vi "calculations.vi"(8 "Jump":dbl format="%#_13g", 10 "Sampling rate":dbl format="%#_13g", 11 "Force data":dbl[](array[numeric])=[2085.326104471059, 2046.9367015003631, 2066.134196083894, 2065.551002863692, 2042.2839241875834, 2031.815973261881, 2023.6720169084117, 2006.8033050654276, 2002.7369130850595, 1985.280219853559, 1978.8890352729054, 1960.2683496851575, 1959.6835604088506, 1957.3819106220842, 1923.0349587901856, 1913.1462109444237, 1900.9278823300624, 1886.9671563075658, 1876.4944172135492, 1866.6040733116827, 1852.0585580128793, 1840.4178364223535, 1822.9627392469579, 1821.2211398668746, 1802.019655143082, 1783.9829608035889, 1772.3446332972203, 1750.2319706407304, 1742.0872162592084, 1722.301740287161, 1696.1178974819888, 1697.8730633389619, 1655.9645503457439, 1664.1364376810463, 1625.7135175321514, 1601.2752642473242, 1582.656174715681, 1558.7971245107942, 1536.692442134828, 1525.0429422357263, 1494.2127063421933, 1479.661604847023, 1444.1642271357675, 1420.8939563474496, 1394.129314406232, 1368.5246746810008, 1342.9248231240833, 1315.573795850454, 1288.8075578531323, 1261.4613187478171, 1230.0375152694012, 1194.5457237545127, 1177.0866364388546, 1145.667621128753, 1111.9166309658945, 1088.6391779251053, 1054.3089846823063, 1023.4715665363022, 992.0461670017816, 964.7015239525717, 942.5976396046577, 910.5874507938302, 876.8284803504483, 851.81421609789, 817.483224827039, 790.1377837497765, 759.297971519615, 735.4413153988853, 706.9223056287473, 681.329636324301, 655.1433994349719, 626.0491767251549, 596.9581461275479, 581.2422542480781, 546.332857925339, 520.7346024245261, 500.3667312603289, 472.4357028787071, 440.43588843256015, 431.1239495825817, 406.10330110560443, 391.5601798909579, 364.20276839291023, 345.0076678935362, 329.87975740258264, 313.003065279075, 292.05838511909434, 278.0928709282835, 259.4673971722215, 243.7586875452231, 229.21077816226247, 213.49648233889715, 203.01895507656647, 178.00309476790346, 165.20396701749735, 156.47681744382552, 144.838489937457, 131.4505827704818, 110.50749866660588, 104.10194958101008, 121.00018846193156, 96.54437855995202, 86.06844735372628, 79.65731207176384, 64.53339172107218, 55.803050035191035, 47.657497625616884, 45.32951291312223, 39.511147187990154, 44.75669405760071, 32.52320291024451, 24.383236697036796, 27.296808713890815, 35.442361123464764, 17.400878615657593, 22.638445204744375, 14.490498711013087, 12.165706110727744, 7.510534713791018, 8.672931013933386, 12.170494279042012, 14.500075047641422, 2.2689779844423468, 12.75049538703473, 6.929735577745719, 4.60095283719889, 6.348138413648245, 5.182550001296365, 8.09612201815018, 11.004905866690132, 1.1041876001426418, 3.4393545651084954, 8.673729041985967, 10.995329530061595, 1.109773796509086, 6.928139521640963, 4.598558753041756, 1.110571824561464, -9.934188096924103, -2.9606083241208556, 2.853767260749333, 7.508140629633681, 12.753687499244243, 1.1113698526138422, 2.855363316853887, -1.2222010562472552, 2.857757401011021, 6.344946301438733, 2.8545652888017115, 5.765743221498595, 7.51292879794795, 3.4377585090039418, 9.843307594599738, -1.2206050001424988, 2.853767260749333, 2.8529692326969553, -1.2190089440379455, 1.1089757684569106, 8.097718074254937, -1.2094326074094082, 1.1089757684569106, 4.021749757258347, 1.6929670167113164, 9.841711538495185, 4.019355673101416, 3.4385565370561175, 4.020153701153592, 4.019355673101416, 3.4385565370561175, 6.344946301438733, 5.759358997079571, 1.6929670167113164, 26.15196903090016, -2.382203272232894, 2.8561613449064676, 4.596962696937, 1.6913709606067628, 4.603346921355822, -0.05421855973824068, 3.4409506212132515, 15.66406740388875, 2.270574040547103, 5.1897322537675645, 1.1025915440378857, 3.436960480951361, 2.855363316853887, 2.852171204644577, -0.05581461584279419, 6.348138413648245, -1.2214030281948771, 5.76654124955077, 2.855363316853887, 1.1081777404045325, 15.669653600255192, 4.603346921355822, 1.1081777404045325, 2.8561613449064676, 1.6905729325543848, 2.8529692326969553, 5.186540141558052, 1.1089757684569106, 5.191328309872321, 20.90562413323742, 1.6905729325543848, 3.4385565370561175, 3.435364424846808, 1.6913709606067628, 2.8561613449064676, 2.271372068599481, 3.4377585090039418, 0.524984520202302, -0.6350176957833369, -0.062198840261819, 1.1065816842997762, -1.2182109159855674, -0.05581461584279419, -0.6374117799404712, -1.2174128879331891, -0.05342053168586258, -34.9971320606764, -0.6374117799404712, 26.148776918690643, -3.5422054882183303, 2.2737661527564126, 4.60015480914631, -0.05421855973824068, 2.276160236913547, 2.8529692326969553, 2.855363316853887, 8.67213298588121, 7.505746545476749, -3.5469936565325986, 15.06890376290105, -4.131782932839585, -1.2174128879331891, 5.181751973243784, -0.05581461584279419, -1.2190089440379455, 2.271372068599481, -1.7998080800830416, 17.994446200540537, 15.654491067260414, 4.020951729206172, 4.020951729206172, 2.272170096651859, 2.8561613449064676, 2.2737661527564126, -0.055016587790618784, 5.767339277603352, 8.676123126142897, -3.544599572375464, 4.014567504787148, -1.802202164240176, -1.2190089440379455, -2.382203272232894, 4.020153701153592, 1.1089757684569106, 1.1113698526138422, -6.451787364810458, -3.5438015443230864, -5.289391064667887, 9.256124234135616, -2.96300240827799, 6.934523746059988, 4.019355673101416, 0.5265805763070582, 5.18334802934854, 3.4377585090039418, 1.6921689886589384, 1.6905729325543848, 7.506544573529127, 2.8561613449064676, 8.678517210300235, -1.8053942764494857, -2.380607216128138, 2.2737661527564126, 3.436960480951361, -0.6358157238357149, -1.7990100520306636, -0.6374117799404712, 0.5257825482546801, 6.926543465536207, -2.3790111600233814, 13.908901546915613, 6.348138413648245, 0.5265805763070582, 4.016961588944282, 2.8545652888017115, 3.436960480951361, 10.416924478173634, -1.2182109159855674, -1.2182109159855674, 6.925745437484031, -16.943679132083755, 0.5289746604639898, -0.05741067194755039, -1.2182109159855674, 5.764945193446015, -11.694142122211304, -2.968588604644434, -0.6334216396785807, 1.6953611008684508, 9.260114374397709, -0.6350176957833369, 4.021749757258347, 8.09133384983591, 1.6921689886589384, 4.019355673101416, 9.837721398233091, 0.5273786043592336, 9.261710430502262, -0.6374117799404712, -5.292583176877197, -5.287795008563131, 1.1089757684569106, 4.019355673101416, -1.8006061081354197, 1.109773796509086, -2.38379932833765, -7.621365917424431, 2.276958264965925, -1.7998080800830416, 4.020153701153592, 4.590578472518178, 0.5265805763070582, 2.8561613449064676, 2.270574040547103, -0.05421855973824068, 5.760955053184326, 0.524984520202302, -1.2182109159855674, 3.4377585090039418, -12.857336450406455, -2.9661945204872997, 1.1089757684569106, -1.2182109159855674, 1.6913709606067628, 0.5289746604639898, -7.618173805214918, 8.680911294457166, -7.6077994405342055, -9.956532882390285, 5.179357889086853, 4.022547785310726, 2.272170096651859, -0.05342053168586258, 4.020951729206172, 2.2737661527564126, 2.8561613449064676, 9.25452817803086, 1.6881788483972504, -0.6350176957833369, -1.215816831828433, -2.380607216128138, -1.2182109159855674, 0.5265805763070582, 0.5289746604639898, 1.6913709606067628, -4.127792792577492, -1.7998080800830416, 9.843307594599738, -0.05581461584279419, 4.603346921355822, -1.2190089440379455, 2.271372068599481, 2.270574040547103, -1.8006061081354197, 1.6937650447636945, 3.4393545651084954, 7.514524854052706, 6.927341493588788, 0.5281766324116117, -6.444605112339257, 0.5257825482546801, 0.5297726885163679, 0.5297726885163679, 1.6921689886589384, 0.5289746604639898, 1.6929670167113164, 5.769733361760283, -3.5438015443230864, -0.055016587790618784, 11.00889600695182, 8.677719182247655, 2.853767260749333, -1.2182109159855674, 1.6929670167113164, 5.761753081236705, -0.05342053168586258, 1.68418870813536, 1.6929670167113164, -2.382203272232894, 9.251336065821754, -6.459767645334036, 5.184146057401121, 2.2753622088611687, 3.4409506212132515, 1.1081777404045325, -7.03737466916962, -2.962204380225612, 22.076798741955745, -2.949435931387765, 15.084864323948409, 2.272170096651859, 2.2737661527564126, 4.60015480914631, -1.2182109159855674, 2.856959372958643, 0.5297726885163679, 10.428096870906522, 2.8545652888017115, -2.3830013002850694, -4.12539870842056, 19.16322672510193, 0.5257825482546801, 1.109773796509086, 1.110571824561464, 3.4377585090039418, 4.021749757258347, -2.382203272232894, 5.184944085453297, 2.853767260749333, 1.1025915440378857, 11.57692669415907, 2.853767260749333, 1.110571824561464, 2.8561613449064676, 4.018557645048835, 2.8585554290633994, 3.436960480951361, -0.6374117799404712, -0.05262250363348448, 5.763349137341258, -4.130186876734829, 3.4385565370561175, 2.270574040547103, 1.6913709606067628, 1.6913709606067628, -3.5469936565325986, -0.6342196677309587, 3.432172312637295, -0.05262250363348448, 14.5008730756938, 15.080874183686518, 15.66406740388875, 22.646425485268153, 32.53916347129166, 43.59908592577221, 52.32862958360097, 56.40699198475469, 72.70767314053133, 86.09238819529702, 131.51043487440893, 153.04150036680116, 150.70074720546867, 183.29732134870807, 218.8034773685396, 260.12720108545045, 306.114076479822, 393.4071189739525, 503.9752204247154, 660.5142367088027, 818.794852372973, 968.9394919641973, 1064.9748465649946, 1098.749777569424, 1076.653075473981, 1010.3174815886691, 913.1205287157817, 826.9771140729557, 746.6568533235761, 658.1806657999416, 612.7785796818771, 597.6498711628711, 602.8850436678008, 637.2056605739712, 671.5214893118275, 709.3308911745303, 723.8700222489149, 708.727747253019, 705.8173673483744, 671.4775977689474, 642.953001802443, 628.3835456620686, 627.7899780771857, 650.4786517014064, 688.8776310087303, 730.191778389013, 778.4978601873033, 840.2022235172494, 859.4172747179323, 901.9177592399285, 936.850298376186, 996.8162544382583, 1003.7842480146951, 1027.053720774961, 1039.2672612210083, 1049.7415963711292, 1062.538330037379, 1049.7296259503441, 1043.895299664165, 1112.5900013560138, 1148.6681782033143, 1185.9135395190717, 1219.6629336258254, 1244.6875722430643, 1265.056241435314, 1275.5329706695923, 1281.357720619143, 1295.9024378898941, 1304.0503843836257, 1320.930268619343, 1333.153385402018, 1370.9699695171923, 1402.3913789114513, 1425.0864367600905, 1447.7814946087303, 1468.7269727967632, 1476.8773133746517, 1503.0619542078764, 1522.2594487914075, 1536.2265590383226, 1550.1936692852385, 1576.9607053106129, 1604.3093385000846, 1647.945086368443, 1693.9072228931914, 1740.457340806456, 1786.4218714153612, 1805.6273462794165, 1825.4104281673065, 1827.73123062733, 1818.9793421840347, 1851.5735222431174, 1856.7791677101093, 1887.6062114914332, 1934.1491471522265, 1987.6760369505043, 2032.4725850629004, 2082.5226603254305, 2109.283312126386, 2124.984041472861, 2135.448002258302, 2128.4480875597706, 2123.201742662108, 2119.120986176797, 2113.8794294474487, 2124.9385538738766, 2130.7569195990086, 2124.358552765884, 2117.379386796714, 2113.324167209079, 2076.0851901177402, 2046.4117643279835, 2016.1679137668618, 1985.918477009374, 1963.2369856376245, 1942.8810848942126, 1939.987463578668, 1917.3067702349704, 1908.5891969979273, 1907.4483474551985, 1857.3847057157782, 1831.7968245796458, 1808.5281498474321, 1788.1674609357062, 1766.058788419478, 1749.1908746045467, 1741.6348996395936, 1734.0781266465879, 1727.683749953725, 1720.1261789326675, 1716.0581908961942, 1706.747050074268, 1693.9479223238618, 1676.4920271204137, 1670.0920642311842, 1663.1097061498049, 1653.220160275991, 1652.6377650838408, 1655.5505390726426, 1656.7209156533086, 1654.9809123293305, 1664.8728522873018, 1656.1401165172638, 1652.068936368581, 1645.0849822310975, 1639.8474156420102, 1647.414562999697, 1639.8410314175912, 1640.426618721951, 1647.9865838271655, 1652.650533532679, 1656.1425106014208, 1648.5673829632108, 1639.2554441132324, 1641.5834288257267, 1641.58103474157, 1635.7642650725425, 1641.0002356055245, 1610.7172816698373]) -> (0 "Peak landing force":dbl, 1 "Peak force":dbl, 2 "flight time":dbl, 3 "Jump height":dbl)   [LabVIEW 2014]
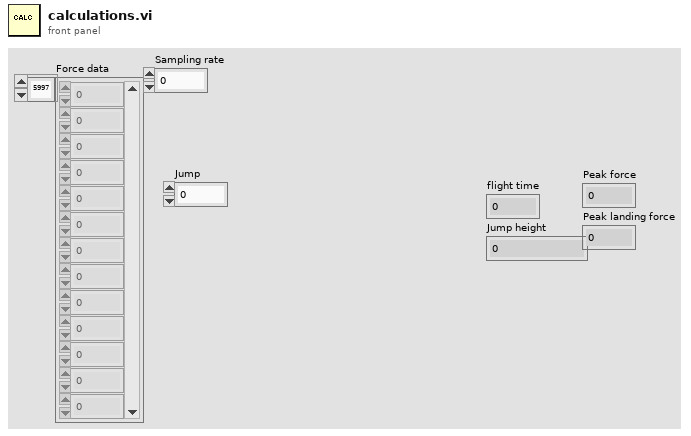
[diagram p1: front panel]
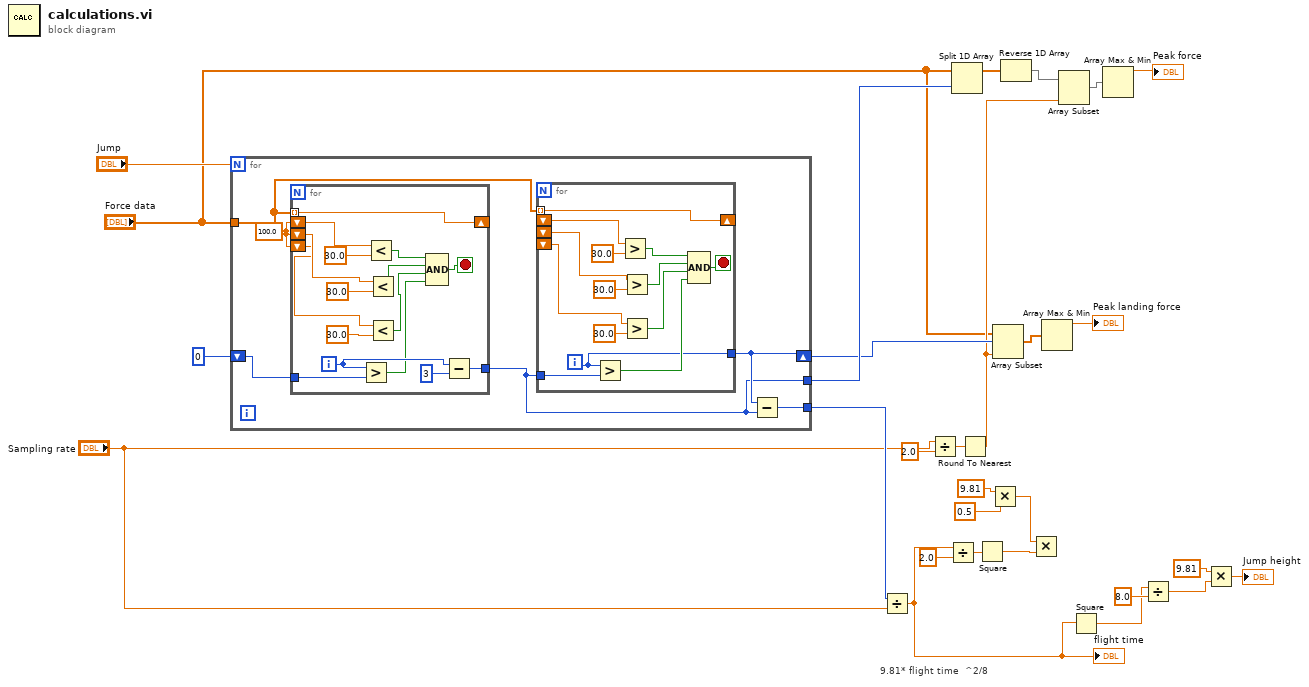
[diagram p0: block diagram]
diagram:
  # "9.81* flight time  ^2/8"
  n1 = for {
    N: "Jump" -> [_]
    tunnel: "Force data" -> [w33]
    tunnel: [w32] -> w28
    shift-right: [w31] -> w23
    shift-left: 0 ("y") -> [w30]
    tunnel: [w29] -> w25
    w34 = 100.0 ("Sample Rate 2")
    n2 = for {
      shift-right: [w64] -> _
      shift-left: w34 -> [w63]
      shift-left: w34 -> [w59]
      shift-left: w34 -> [w58]
      tunnel: w33 -> [w64] mode=indexing
      tunnel: [w52] -> w29
      tunnel: w30 -> [w50]
      i -> [w51]
      stop <- w54 stop-if-true
      n3 = Greater?(x=w51, y=w50) -> (0:w49:bool)
      n4 = Less?(x=w63, y=30.0) -> (x < y?=w57:bool)
      n5 = Less?(x=w59, y=30.0) -> (x < y?=w56:bool)
      n6 = Less?(x=w58, y=30.0) -> (x < y?=w55:bool)
      n7 = Compound Arithmetic op=AND(w57, w56, w55, w49) -> (w54:bool)
      n8 = Subtract(x=w51, y=3) -> (x-y=w52:i32)
    }
    n9 = for {
      shift-right: [w48] -> _
      shift-left: _ -> [w47]
      shift-left: _ -> [w43]
      shift-left: _ -> [w42]
      tunnel: w33 -> [w48] mode=indexing
      tunnel: w29 -> [w37]
      tunnel: [w35] -> w31
      i -> [w35]
      stop <- w38 stop-if-true
      n10 = Greater?(x=w35, y=w37) -> (0:w36:bool)
      n11 = Greater?(x=w47, y=30.0) -> (0:w41:bool)
      n12 = Greater?(x=w43, y=30.0) -> (0:w40:bool)
      n13 = Greater?(x=w42, y=30.0) -> (0:w39:bool)
      n14 = Compound Arithmetic op=AND(w41, w40, w39, w36) -> (w38:bool)
    }
    n15 = Subtract(x=w31, y=w29) -> (x-y=w32:i32)
  }
  n16 = Divide(x=w28, y="Sampling rate") -> (x/y=w2:dbl)
  "flight time" <- w2
  n17 = Divide(x="Sampling rate", y=2.0) -> (x/y=w20:dbl)
  n18 = Divide(x=w2, y=2.0) -> (x/y=w9:dbl)
  n19 = Split 1D Array(array="Force data", index=w25) -> (first subarray=w24:dbl[])  [unwired: 1 out]
  n20 = Round To Nearest(number=w20) -> (nearest integer value=w16:dbl)
  n21 = Square(x=w9) -> (x^2=w7:dbl)
  n22 = Multiply(x=9.81, y=0.5) -> (x*y=w8:dbl)
  n23 = Array Subset(array="Force data", index=w23, length=w16) -> (w19:dbl[])
  n24 = Reverse 1D Array(array=w24) -> (reversed array=w17:dbl[])
  n25 = Multiply(x=w8, y=w7) -> ()  [unwired: 1 out]
  n26 = Array Max & Min(array=w19) -> (max value=→"Peak landing force":dbl)  [unwired: 3 out]
  n27 = Array Subset(array=w17, length=w16) -> (w15:dbl[])  [unwired: 1 in]
  n28 = Square(x=w2) -> (x^2=w4:dbl)
  n29 = Array Max & Min(array=w15) -> (max value=→"Peak force":dbl)  [unwired: 3 out]
  n30 = Divide(x=w4, y=8.0) -> (x/y=w3:dbl)
  n31 = Multiply(x=9.81, y=w3) -> (x*y=→"Jump height":dbl)
